vi "MB Decode Data.vi"(7 "Quantity":u16, 8 "error in (no error)":errorcluster, 10 "Response MDU":T1={"function"=1, "Data"=[]} {"function" items=["Read Discrete Inputs"=2, "Read Coils"=1, "Write Single Coil"=5, "Write Multiple Coils"=15, "Read Input Register"=4, "Read Holding Registers"=3, "Write Single Register"=6, "Write Multiple Registers"=16, "Read/Write Multiple Registers"=23, "Mask Write Register"=22, "Read FIFO Queue"=24, "Read File Record"=20, "Write File Record"=21, "Read Exception Status"=7, "Diagnostic"=8, "Get Com Event Counter"=11, "Get Com Event Log"=12, "Report Slave ID"=17, "Read Device Identification"=43]; "Data" format="%.0x"}, 11 "Function Code":u8) -> (0 "error out":errorcluster, 2 "Discrete":bool[](array[boolean]), 3 "Registers":u16[](array[numeric]))   [LabVIEW 2019, in "NI_modbus_upd.lvlib"]
uses:
  NI_modbus_upd.lvlib
  Ctl/MB Modbus Data Unit.ctl
  Modbus Data Unit (PDU)/Function.ctl
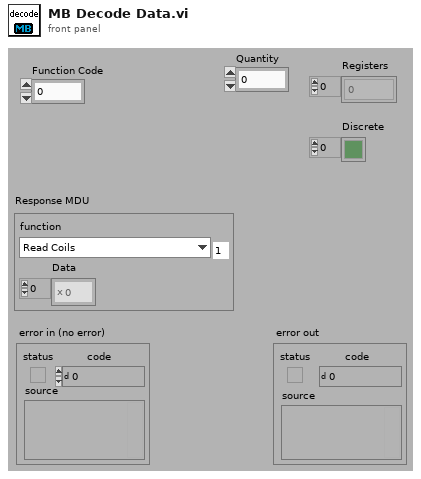
[diagram p1: front panel]
types:
  T1 = typedef "NI_modbus_upd.lvlib/MB Modbus Data Unit.ctl" = cluster{"function":T2, "Data":u8[]}
  T2 = typedef "NI_modbus_upd.lvlib/Function.ctl" = u8
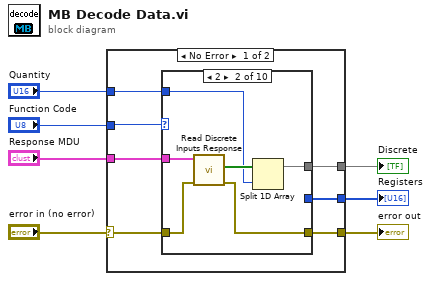
[diagram p0: block diagram]
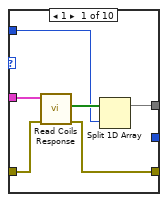
[diagram p2: hidden frame]
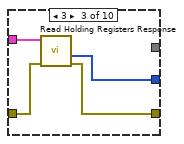
[diagram p3: hidden frame]
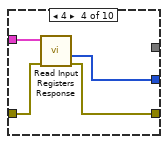
[diagram p4: hidden frame]
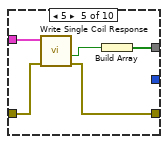
[diagram p5: hidden frame]
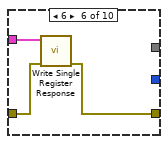
[diagram p6: hidden frame]
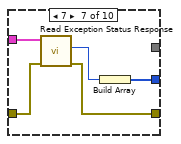
[diagram p7: hidden frame]
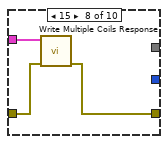
[diagram p8: hidden frame]
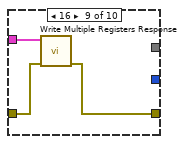
[diagram p9: hidden frame]
diagram:
  n1 = case shown="No Error" "error in (no error)" {
    selector: "error in (no error)" -> [w11 w55]
    tunnel: "Response MDU" -> [w12 _]
    tunnel: [w14 _] -> w6
    tunnel: [w13 _] -> w5
    tunnel: "Function Code" -> [w8 _]
    tunnel: [w10 w55] -> w3
    tunnel: "Quantity" -> [w9 _]
    frame No Error {
      n2 = case shown="2" w8 {
        tunnel: [w16 w22 _ _ w37 _ _ _ _ _] -> w14
        tunnel: [_ _ w29 w33 _ _ w45 _ _ _] -> w13
        tunnel: w12 -> [w20 w26 w30 w34 w39 w42 w47 w50 w53 _]
        tunnel: w11 -> [w19 w25 w28 w32 w36 w41 w44 w49 w52 w54]
        tunnel: [w18 w24 w27 w31 w35 w40 w43 w48 w51 w54] -> w10
        tunnel: w9 -> [w15 w21 _ _ _ _ _ _ _ _]
        frame 1 {
          n3 = call "Read Coils Response.vi"("error in (no error)"=w19, 11:w20) -> ("error out"=w18:errorcluster, "data"=w17:bool[])  [unwired: 8 in]
          n4 = Split 1D Array(array=w17, index=w15) -> (first subarray=w16:bool[])  [unwired: 1 out]
        }
        frame 2 {
          n5 = call "Read Discrete Inputs Response.vi"("error in (no error)"=w25, 11:w26) -> ("error out"=w24:errorcluster, "data"=w23:bool[])  [unwired: 8 in]
          n6 = Split 1D Array(array=w23, index=w21) -> (first subarray=w22:bool[])  [unwired: 1 out]
        }
        frame 3 {
          n7 = call "Read Holding Registers Response.vi"("error in (no error)"=w28, 11:w30) -> ("error out"=w27:errorcluster, "register values"=w29:u16[])  [unwired: 7 in, 1 out]
        }
        frame 4 {
          n8 = call "Read Input Registers Response.vi"("error in (no error)"=w32, 11:w34) -> ("error out"=w31:errorcluster, "register values"=w33:u16[])  [unwired: 7 in, 1 out]
        }
        frame 5 {
          n9 = call "Write Single Coil Response.vi"("error in (no error)"=w36, 11:w39) -> ("error out"=w35:errorcluster, "coil value"=w38:bool)  [unwired: 7 in, 1 out]
          n10 = Build Array(w38) -> (w37:bool[])
        }
        frame 6 {
          n11 = call "Write Single Register Response.vi"("error in (no error)"=w41, 11:w42) -> ("error out"=w40:errorcluster)  [unwired: 7 in, 2 out]
        }
        frame 7 {
          n12 = call "Read Exception Status Response.vi"("error in (no error)"=w44, 11:w47) -> ("error out"=w43:errorcluster, "exception status"=w46:u8)  [unwired: 8 in]
          n13 = Build Array(w46) -> (w45:u8[])
        }
        frame 15 {
          n14 = call "Write Multiple Coils Response.vi"("error in (no error)"=w49, 11:w50) -> ("error out"=w48:errorcluster)  [unwired: 7 in, 2 out]
        }
        frame 16 {
          n15 = call "Write Multiple Registers Response.vi"("error in (no error)"=w52, 11:w53) -> ("error out"=w51:errorcluster)  [unwired: 7 in, 2 out]
        }
        frame Default {
        }
      }
    }
    frame Error {
    }
  }
  "error out" <- w3
  "Registers" <- w5
  "Discrete" <- w6
